vi "sort channels.vi"(8 "error in (no error)":errorcluster, 11 "channels in":refnum<class "TBM channel.lvclass">[](array[class])) -> (0 "error out":errorcluster, 3 "channels out":refnum<class "TBM channel.lvclass">[](array[class]))   [LabVIEW 2013, in "Shared Memory configuration.lvclass"]
uses:
  module/configuration/Shared Memory configuration.lvclass
  <vilib>/NI/Tag Bus Module Framework/channel/TBM channel.lvclass
  <vilib>/NI/Tag Bus/tag/Data Type.ctl
  <vilib>/NI/Tag Bus/tag/tag descriptor.lvclass/tag descriptor.ctl
  <vilib>/NI/Tag Bus/tag/tag descriptor.lvclass
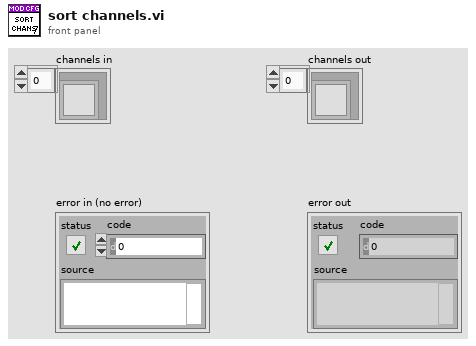
[diagram p1: front panel]
types:
  T1 = typedef "tag bus.lvlib/tag descriptor.lvclass/Data Type.ctl" = enum16{"Double", "Single", "I64", "I32", "I16", "I8", "U64", "U32", "U16", "U8", "Boolean", "String", "Array of Double", "Array of Single", "Array of I64", "Array of I32", "Array of I16", "Array of I8", "Array of U64", "Array of U32", "Array of U16", "Array of U8", "Array of Boolean", "Array of String"}
  T2 = cluster{"name":string, "system tag out":refnum<class "TBM channel.lvclass">}
  T3 = cluster{"name":string, "system tag out":refnum<class "TBM channel.lvclass">}[]
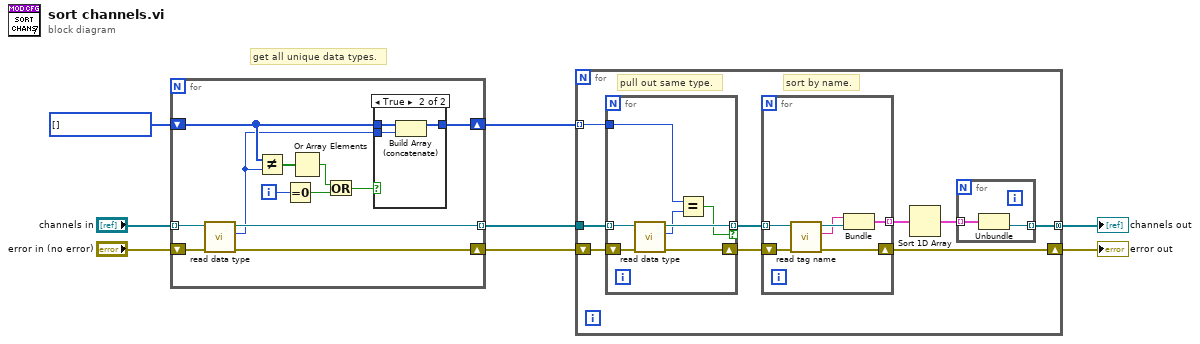
[diagram p0: block diagram]
diagram:
  w7 = T1[] [] items=["Double", "Single", "I64", "I32", "I16", "I8", "U64", "U32", "U16", "U8", "Boolean", "String", "Array of Double", "Array of Single", "Array of I64", "Array of I32", "Array of I16", "Array of I8", "Array of U64", "Array of U32", "Array of U16", "Array of U8", "Array of Boolean", "Array of String"]
  # "get all unique data types."
  n1 = for {
    tunnel: "channels in" -> [w20] mode=indexing
    shift-right: [w18] -> w5
    shift-left: w7 -> [w17]
    shift-right: [w12] -> w3
    shift-left: "error in (no error)" -> [w11]
    tunnel: [w10] -> w4 mode=indexing
    i -> [w19]
    n2 = call <vilib>:"read data type.vi"("error in"=w11, "system tag in"=w20) -> ("error out"=w12:errorcluster, "data type"=w9:T1, "system tag out"=w10:refnum<class "TBM channel.lvclass">)  [unwired: 7 in]
    n3 = Not Equal?(x=w17, y=w9) -> (x != y?=w16:bool[])
    n4 = Equal To 0?(x=w19) -> (x = 0?=w14:bool)
    n5 = Or Array Elements(Boolean array=w16) -> (logical OR=w15:bool)
    n6 = Or(x=w15, y=w14) -> (x .or. y?=w13:bool)
    n7 = case shown="True" w13 {
      tunnel: w17 -> [w21 w24]
      tunnel: [w21 w23] -> w18
      tunnel: w9 -> [_ w22]
      frame False {
      }
      frame True {
        n8 = Build Array (concatenate)(w24, w22) -> (w23:T1[])
      }
    }
  }
  n9 = for {
    tunnel: w5 -> [w31] mode=indexing
    tunnel: w4 -> [w33]
    shift-right: [w27] -> w1
    shift-left: w3 -> [w32]
    tunnel: [w25] -> w2 mode=concatenating
    # "sort by name."
    # "pull out same type."
    n10 = for {
      tunnel: w33 -> [w48] mode=indexing
      shift-right: [w46] -> w30
      shift-left: w32 -> [w47]
      tunnel: w31 -> [w45]
      tunnel: [w44] -> w29 mode=indexing if=w42
      n11 = call <vilib>:"read data type.vi"("error in"=w47, "system tag in"=w48) -> ("error out"=w46:errorcluster, "data type"=w43:T1, "system tag out"=w44:refnum<class "TBM channel.lvclass">)  [unwired: 7 in]
      n12 = Equal?(x=w45, y=w43) -> (x = y?=w42:bool)
    }
    n13 = for {
      tunnel: w29 -> [w41] mode=indexing
      shift-right: [w39] -> w27
      shift-left: w30 -> [w40]
      tunnel: [w36] -> w28 mode=indexing
      n14 = call <vilib>:"read tag name.vi"("error in"=w40, "system tag in"=w41) -> ("error out"=w39:errorcluster, "name"=w37:string, "system tag out"=w38:refnum<class "TBM channel.lvclass">)  [unwired: 7 in]
      n15 = Bundle("name"=w37, "system tag out"=w38) -> (w36:T2)  [unwired: 1 in]
    }
    n16 = Sort 1D Array(array=w28) -> (sorted array=w26:T3)
    n17 = for {
      tunnel: w26 -> [w35] mode=indexing
      tunnel: [w34] -> w25 mode=indexing
      n18 = Unbundle(w35) -> ("system tag out"=w34:refnum<class "TBM channel.lvclass">)  [unwired: 1 out]
    }
  }
  "channels out" <- w2
  "error out" <- w1
